vi "Lockin.DAQ.Start.AO.vi"(8 "error in (no error)":errorcluster, 11 "Lockin.DAQ in":refnum<class "Lockin.DAQ.lvclass">) -> (0 "error out":errorcluster, 3 "Lockin.DAQ out":refnum<class "Lockin.DAQ.lvclass">)   [LabVIEW 2016, in "Lockin.DAQ.lvclass"]
uses:
  Lockin.DAQ.lvclass
  Lockin.DAQ.lvclass/Lockin.DAQ.ctl
  <vilib>/DAQmx/write.llb/DAQmx Write (Analog 1D Wfm NChan NSamp).vi
  <vilib>/DAQmx/miscellaneous.llb/DAQmx Fill In Error Info.vi
panel:
  out "reset indicator":bool
  out "Array":u32[](array[numeric])
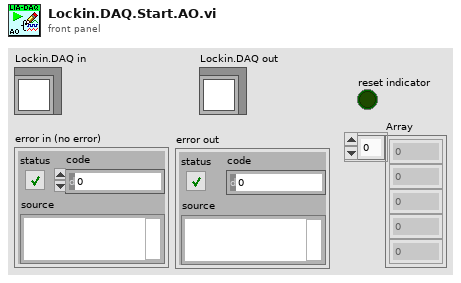
[diagram p1: front panel]
types:
  T1 = typedef "Lockin.DAQ.lvclass/DAQType-enum.ctl" = enum16{"None", "USB 4431", "PXI 446x"}
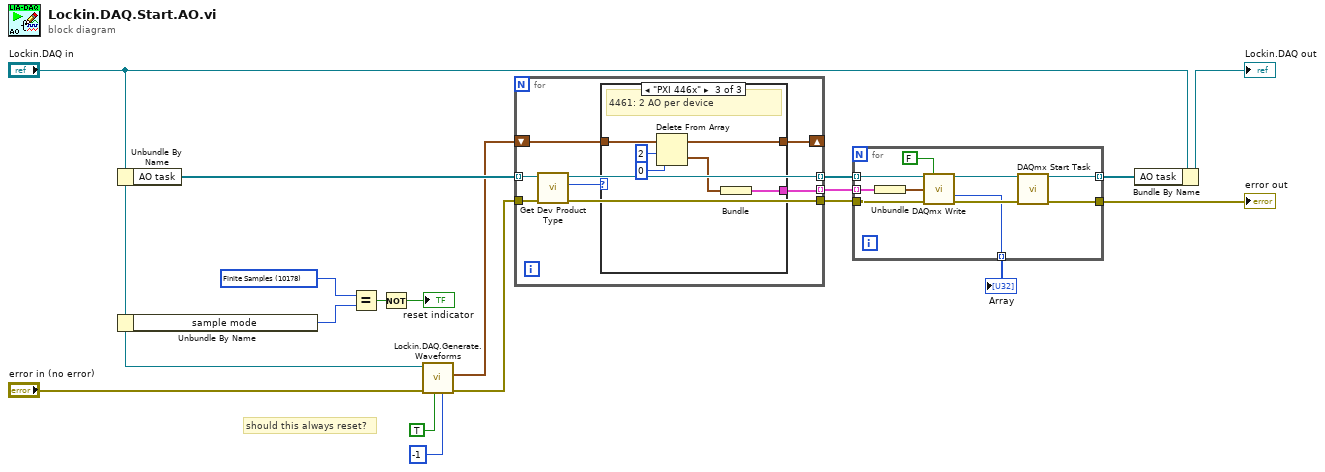
[diagram p0: block diagram]
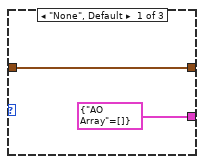
[diagram p2: hidden frame]
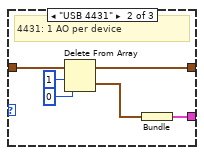
[diagram p3: hidden frame]
diagram:
  w3 = 10178 items=["Finite Samples"=10178, "Continuous Samples"=10123] ("sample mode 2")
  # "should this always reset?"
  n1 = Unbundle By Name("Lockin.DAQ in") -> ("AO task"=w14:refnum<k21>[])
  n2 = Unbundle By Name("Lockin.DAQ in") -> ("sample mode"=w2:i32)
  n3 = Equal?(x=w3, y=w2) -> (x = y?=w18:bool)
  n4 = Not(x=w18) -> (.not. x?=→"reset indicator":bool)
  n5 = call "Lockin.DAQ.Generate.Waveforms.vi"("sweep index"=-1, "Reset?"=TRUE ("reset signal"), "error in (no error)"="error in (no error)", "Lockin.DAQ"="Lockin.DAQ in") -> ("error out"=w6:errorcluster, "AO []"=w7:waveform(dbl)[])  [unwired: 3 in, 3 out]
  n6 = for {
    tunnel: w14 -> [w26] mode=indexing
    shift-right: [w24] -> _
    shift-left: w7 -> [w25]
    tunnel: [w23] -> w13 mode=indexing
    tunnel: [w22] -> w12 mode=indexing
    tunnel: w6 -> [w21]
    tunnel: [w20] -> w11
    n7 = call "Get Dev Product Type.vi"("error in (no error)"=w21, "Refnum in"=w26) -> ("error out"=w20:errorcluster, "DAQ Type"=w19:T1, "Refnum out"=w22:refnum<k21>)  [unwired: 6 in, 1 out]
    n8 = case shown="\"PXI 446x\"" w19 {
      tunnel: w25 -> [w28 w34 w40]
      tunnel: [w28 w33 w39] -> w24
      tunnel: [cluster{"AO Array":waveform(dbl)[]} {"AO Array"=[]} w31 w36] -> w23
      frame "None", Default {
      }
      frame "USB 4431" {
        # "4431: 1 AO per device"
        n9 = Delete From Array(array=w34, length=1, index=0) -> (deleted portion=w30:waveform(dbl)[], array with subset deleted=w33:waveform(dbl)[])
        n10 = Bundle("AO []"=w30) -> (w31:cluster{"AO []":waveform(dbl)[]})  [unwired: 1 in]
      }
      frame "PXI 446x" {
        # "4461: 2 AO per device"
        n11 = Delete From Array(array=w40, length=2, index=0) -> (deleted portion=w37:waveform(dbl)[], array with subset deleted=w39:waveform(dbl)[])
        n12 = Bundle("AO []"=w37) -> (w36:cluster{"AO []":waveform(dbl)[]})  [unwired: 1 in]
      }
    }
  }
  n13 = for {
    tunnel: w12 -> [w48] mode=indexing
    tunnel: w11 -> [w47]
    tunnel: [w46] -> w15
    tunnel: [w45] -> w16 mode=indexing
    tunnel: w13 -> [w44] mode=indexing
    tunnel: [w41] -> w10 mode=indexing
    n14 = Unbundle(w44) -> ("AO []"=w43:waveform(dbl)[])
    n15 = call-poly <vilib>:"DAQmx Write.vi"("task/channels in"=w48, "auto start"=FALSE, "data"=w43, "error in"=w47) -> ("task out"=w49:refnum<k21>, "number of samples written per channel"=w41:u32, "error out"=w50:errorcluster)  [unwired: 9 in]
    n16 = call <vilib>:"DAQmx Start Task.vi"("task/channels in"=w49, "error in"=w50) -> ("task out"=w45:refnum<k21>, "error out"=w46:errorcluster)  [unwired: 12 in]
  }
  "error out" <- w15
  "Array" <- w10
  n17 = Bundle By Name(cluster="Lockin.DAQ in", "AO task"=w16) -> (→"Lockin.DAQ out":refnum<class "Lockin.DAQ.lvclass">)
